vi "rmSharedMemory.vi"(8 "error in (no error)":errorcluster, 10 "nameCsc":string, 11 "TestProcess in":refnum<class "TestProcess.lvclass">) -> (0 "error out":errorcluster, 2 "outputMsg":string, 3 "TestProcess out":refnum<class "TestProcess.lvclass">)   [LabVIEW 2018, in "TestProcess.lvclass"]
doc: "Remove the shared memory of commandable SAL component (CSC)."
uses:
  TestProcess.lvclass
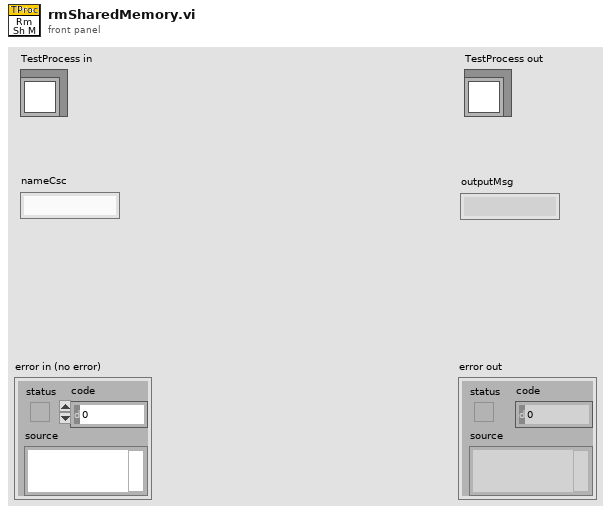
[diagram p1: front panel]
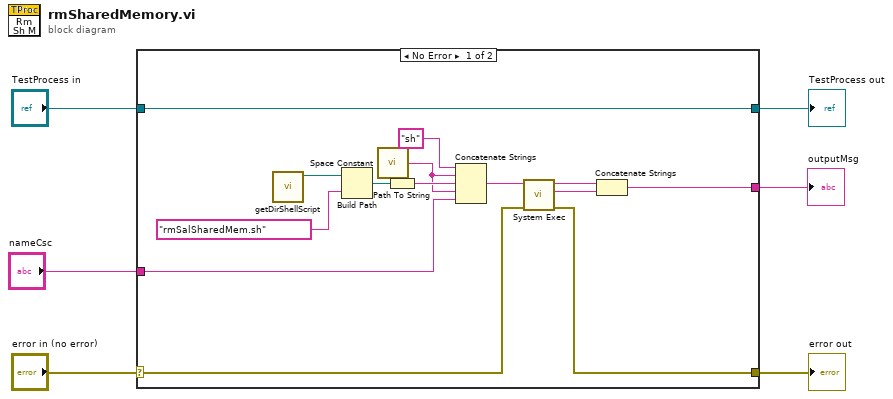
[diagram p0: block diagram]
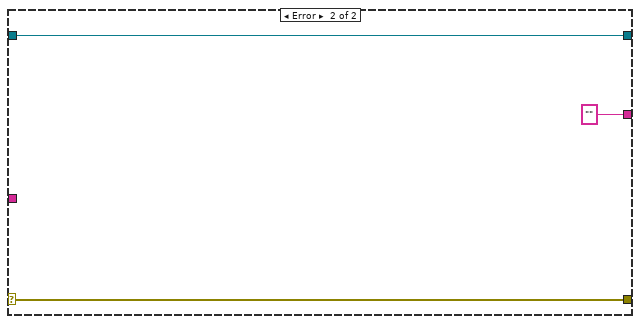
[diagram p2: hidden frame]
diagram:
  n1 = case shown="No Error" "error in (no error)" {
    selector: "error in (no error)" -> [w14 w23]
    tunnel: [w13 w23] -> w5
    tunnel: [w20 w22] -> w3
    tunnel: "TestProcess in" -> [w20 w22]
    tunnel: "nameCsc" -> [w15 _]
    tunnel: [w7 ""] -> w1
    frame No Error {
      n2 = call "getDirShellScript.vi"() -> ("dirShellScript"=w19:path)  [unwired: 11 in]
      n3 = Build Path(base path=w19, name or relative path="rmSalSharedMem.sh") -> (appended path=w17:path)
      n4 = call <vilib>:"Space Constant.vi"() -> ("String"=w12:string)
      n5 = Path To String(path=w17) -> (string=w16:string)
      n6 = Concatenate Strings("sh" ("string"), w12, w16, w12, w15) -> (w10:string)
      n7 = call <vilib>:"System Exec.vi"("error in (no error)"=w14, "command line"=w10) -> ("error out"=w13:errorcluster, "standard error"=w8:string, "standard output"=w9:string)  [unwired: 6 in, 1 out]
      n8 = Concatenate Strings(w9, w8) -> (w7:string)
    }
    frame Error {
    }
  }
  "error out" <- w5
  "TestProcess out" <- w3
  "outputMsg" <- w1
